vi "test.vi"   [LabVIEW 2012]
uses:
  <userlib>/cvlib/cvlib.lvlib
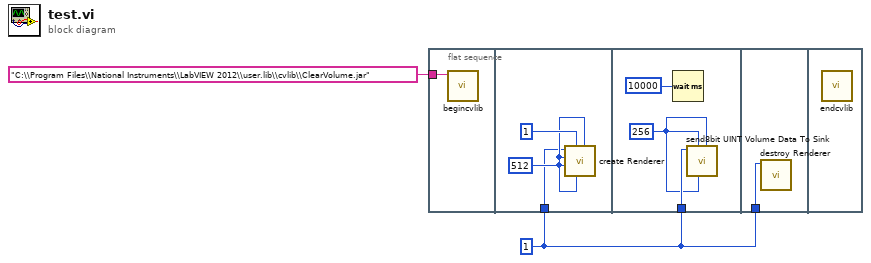
[diagram p0: block diagram]
diagram:
  w1 = 1 ("pRendererId")
  n1 = flat-sequence {
    tunnel: "C:\\Program Files\\National Instruments\\LabVIEW 2012\\user.lib\\cvlib\\ClearVolume.jar" ("AutoPilotJarPath") -> [w3]
    tunnel: w1 -> [w4]
    tunnel: w1 -> [w8]
    tunnel: w1 -> [w10]
    frame #0 {
      n2 = call <userlib>:"begincvlib.vi"("AutoPilotJarPath"=w3) -> ()  [unwired: 9 in, 2 out]
    }
    frame #1 {
      w5 = 512 ("pWindowWidth")
      n3 = call <userlib>:"create Renderer.vi"("pMaxTextureHeight"=w5, "pMaxTextureWidth"=w5, "pBytesPerVoxel"=1, "pWindowHeight"=w5, "pWindowWidth"=w5, "pRendererId"=w4) -> ()  [unwired: 5 in, 1 out]
    }
    frame #2 {
      w7 = 256 ("pRendererId")
      n4 = Wait (ms)(milliseconds to wait=u32 10000) -> ()  [unwired: 1 out]
      n5 = call <userlib>:"send8bit UINT Volume Data To Sink.vi"("pDepthInVoxels"=w7, "pHeightInVoxels"=w7, "pWidthInVoxels"=w7, "pSinkId"=w8) -> ()  [unwired: 6 in, 2 out]
    }
    frame #3 {
      n6 = call <userlib>:"destroy Renderer.vi"("pRendererId"=w10) -> ()  [unwired: 10 in, 1 out]
    }
    frame #4 {
      n7 = call <userlib>:"endcvlib.vi"() -> ()  [unwired: 11 in, 1 out]
    }
  }
